vi "ADS1115_READ_N_SAMPLE_STREAMING.vi"(6 "options_i2c_read":T1, 8 "error in (no error)":errorcluster, 9 "Scale Value (mV)":dbl=2.0, 10 "I2C Slave Address (0)":u8, 11 "handle":u32) -> (0 "error out":errorcluster, 2 "Data read":u8[](array[numeric]) format="%.0x", 3 "handle out":u32)   [LabVIEW 2017]
uses:
  libMPSSE.lvlib
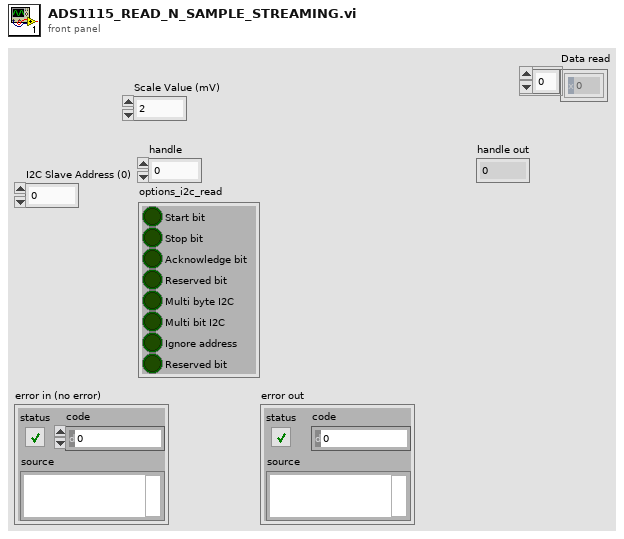
[diagram p1: front panel]
types:
  T1 = cluster{"Start bit":bool, "Stop bit":bool, "Acknowledge bit":bool, "Reserved bit":bool, "Multi byte I2C":bool, "Multi bit I2C":bool, "Ignore address":bool, "Reserved bit":bool}
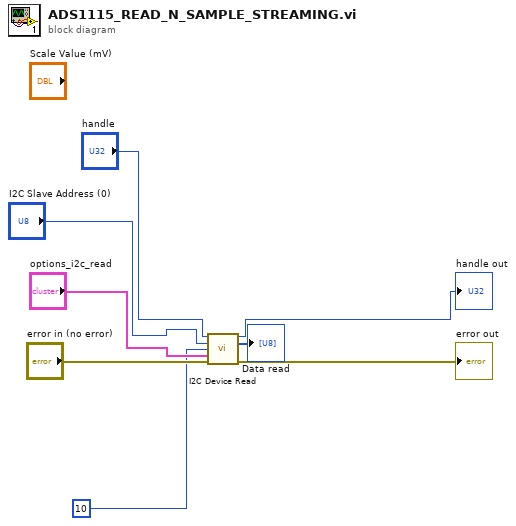
[diagram p0: block diagram]
diagram:
  n1 = call "I2C Device Read.vi"("handle"="handle", "Slave device address"="I2C Slave Address (0)", "Size to transfer"=u32 10 ("N_Samples"), "options"="options_i2c_read", "error in (no error)"="error in (no error)") -> ("handle out"=→"handle out":u32, "Data read"=→"Data read":u8[], "error out"=→"error out":errorcluster)  [unwired: 6 in, 2 out]
